vi "Execute-action.vi"(8 "error in (no error)":errorcluster, 11 "Object ref in":T1) -> (0 "error out":errorcluster, 3 "Object ref out":T1)   [LabVIEW 2013, in "PowderDeposition.lvlib" / "PD-Main.lvclass"]
uses:
  PD-Main.lvclass
  Object-reference.ctl
  PD-Main.lvclass/PD-Main.ctl
  Custom-errors.ctl
  Action/Action.lvclass
  Read Motor assembly.vi
  Read Selected motor.vi
  Read Sequence index.vi
  Assembly/Motor-assembly.lvclass
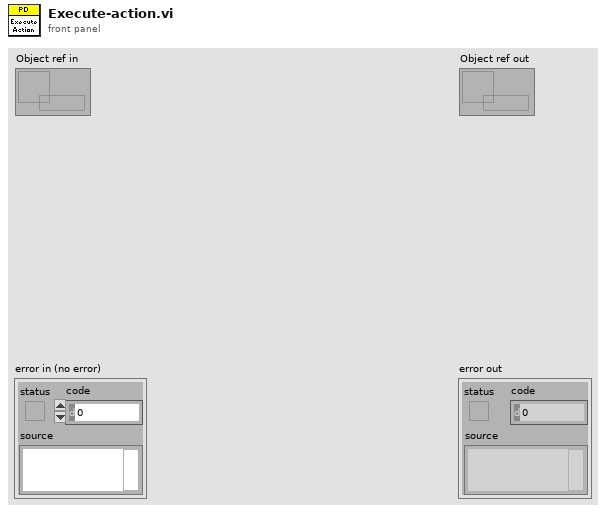
[diagram p1: front panel]
types:
  T1 = typedef "PowderDeposition.lvlib/PD-Main.lvclass/Object-reference.ctl" = refnum<data-value>
  T2 = typedef "PowderDeposition.lvlib/PD-Main.lvclass/Custom-errors.ctl" = enum16{"Not implemented", "Command not recognized", "Invalid input", "Timeout", "Load file failed", "Action failed", "Action invalid", "Motor inactive", "Not in range", "Unsafe state"}
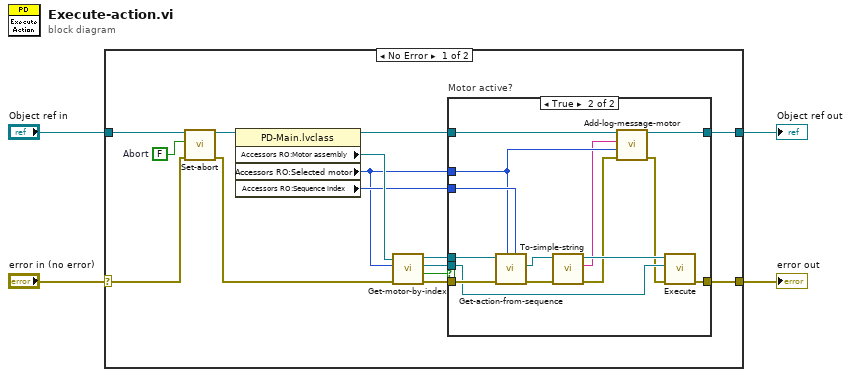
[diagram p0: block diagram]
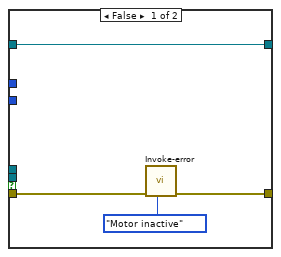
[diagram p2: hidden frame]
diagram:
  n1 = case shown="No Error" "error in (no error)" {
    selector: "error in (no error)" -> [w6 w38]
    tunnel: [w11 w38] -> w3
    tunnel: [w10 w37] -> w1
    tunnel: "Object ref in" -> [w8 w37]
    frame No Error {
      w9 = FALSE  # Abort
      n2 = call "Set-abort.vi"("error in (no error)"=w6, "Abort"=w9, "Object ref in"=w8) -> ("error out"=w5:errorcluster, "Object ref out"=w7:T1)  [unwired: 7 in]
      n3 = property class="PD-Main.lvclass"(reference=w7) -> (reference out=w13:T1, "Accessors RO:Motor assembly"=w15:refnum<class "Motor-assembly.lvclass">, "Accessors RO:Selected motor"=w12:i32, "Accessors RO:Sequence index"=w14:i32)  [unwired: 1 in, 1 out]
      n4 = call "Get-motor-by-index.vi"("error in (no error)"=w5, "Index"=w12, "Available motors in"=w15) -> ("error out"=w19:errorcluster, "Active?"=w16:bool, "Motor"=w18:refnum<class "Motor.lvclass">, "Available motors out"=w17:refnum<class "Motor-assembly.lvclass">)  [unwired: 5 in]
      n5 = case "Motor active?" shown="True" w16 {
        tunnel: w12 -> [_ w31]
        tunnel: w19 -> [w22 w36]
        tunnel: w14 -> [_ w35]
        tunnel: w18 -> [_ w30]
        tunnel: w17 -> [_ w34]
        tunnel: [w21 w24] -> w11
        tunnel: [w23 w33] -> w10
        tunnel: w13 -> [w23 w32]
        frame False {
          n6 = call "Invoke-error.vi"("Error"=Custom-errors."Motor inactive", "error in (no error)"=w22) -> ("error out"=w21:errorcluster)  [unwired: 9 in]
        }
        frame True {
          n7 = call "Get-action-from-sequence.vi"("Sequence index in"=w35, "Motor index"=w31, "error in (no error)"=w36, "Available motors in"=w34) -> ("error out"=w27:errorcluster, "Action"=w29:refnum<class "Action.lvclass">)  [unwired: 4 in, 2 out]
          n8 = call-dynamic "To-simple-string.vi"("error in (no error)"=w27, "Action in"=w29) -> ("error out"=w26:errorcluster, "Action string"=w28:string)  [unwired: 7 in, 1 out]
          n9 = call "Add-log-message-motor.vi"("error in (no error)"=w26, "Motor index"=w31, "Message"=w28, "UI in"=w32) -> ("error out"=w25:errorcluster, "UI out"=w33:T1)  [unwired: 6 in]
          n10 = call-dynamic "Execute.vi"("error in (no error)"=w25, "Motor in"=w30, "Action in"=w29) -> ("error out"=w24:errorcluster)  [unwired: 5 in, 3 out]
        }
      }
    }
    frame Error {
    }
  }
  "error out" <- w3
  "Object ref out" <- w1
